vi "Re-Start Measurement.vi"(8 "error in (no error)":errorcluster, 11 "Spectrum Recorder too in":refnum<class "Spectrum Recorder too.lvclass">) -> (0 "error out":errorcluster, 3 "Spectrum Recorder too out":refnum<class "Spectrum Recorder too.lvclass">)   [LabVIEW 2018, in "Spectrum Recorder too.lvclass"]
uses:
  Spectrum Recorder too.lvclass
  C:/github/2018/LabActor/Instrument Actor/Instrument Actor.lvclass
  Spectrum Recorder too.lvclass/Spectrum Recorder too.ctl
  Instrument Actor/Instrument Actor.lvclass/Instrument Actor.ctl
  Instrument Actor/Read Instrument driver.vi
  Instrument Actor/Write Instrument driver.vi
  NHMFL_Core/Libraries/Instruments/Instrument Driver/Instrument Driver.lvclass
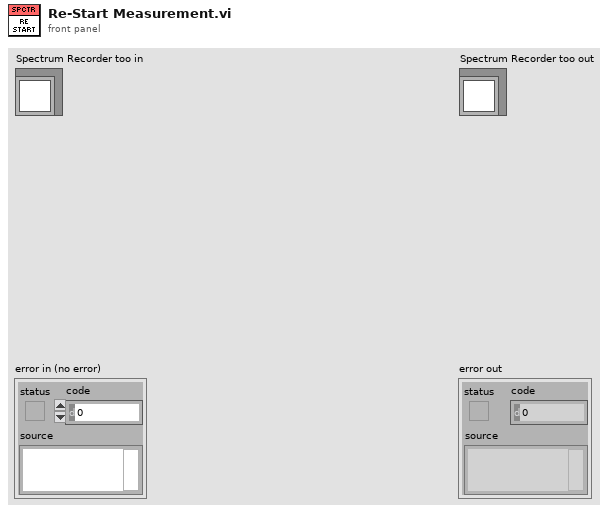
[diagram p1: front panel]
types:
  T1 = enum16{"open", "replace", "create", "open or create", "replace or create", "replace or create with confirmation"}
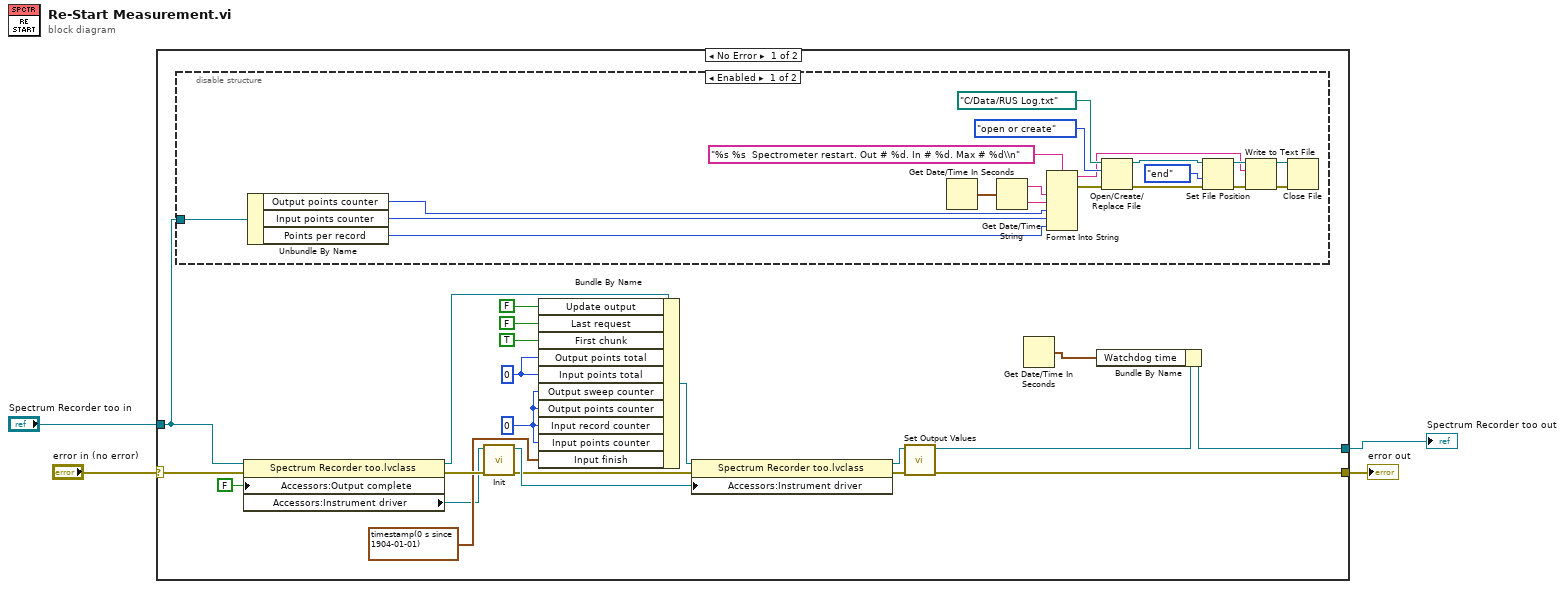
[diagram p0: block diagram]
diagram:
  n1 = case shown="No Error" "error in (no error)" {
    selector: "error in (no error)" -> [w15 w46]
    tunnel: [w10 w46] -> w3
    tunnel: [w6 w45] -> w1
    tunnel: "Spectrum Recorder too in" -> [w7 w45]
    frame No Error {
      w20 = i64 0 ("Output points total")
      w18 = 0 ("Output sweep counter")
      n2 = disable-structure shown="Enabled" {
        disable-tunnel: w7 -> [w29 _]
        frame Enabled {
          n3 = Unbundle By Name(w29) -> ("Output points counter"=w28:i32, "Input points counter"=w27:i32, "Points per record"=w26:i32)
          n4 = Get Date/Time In Seconds() -> (seconds since 1Jan1904=w34:timestamp)
          n5 = Get Date/Time String(seconds (now)=w34) -> (date string=w33:string, time string=w32:string)  [unwired: 2 in]
          n6 = Format Into String(format string="%s %s  Spectrometer restart. Out # %d. In # %d. Max # %d\\n", w33, w32, w28, w27, w26) -> (resulting string=w31:string, error out=w30:errorcluster)  [unwired: 2 in]
          n7 = Open/Create/Replace File(file path (use dialog)=path "C:/Data/RUS Log.txt" ("file (use dialog)"), error in=w30, operation (0:open)=T1."open or create") -> (refnum out=w42:refnum<file>, error out=w39:errorcluster)  [unwired: 3 in, 1 out]
          n8 = Set File Position(refnum=w42, from (0:start)=enum16{"start", "end", "current"}."end", error in=w39) -> (refnum out=w41:refnum<file>, error out=w38:errorcluster)  [unwired: 1 in]
          n9 = Write to Text File(file (use dialog)=w41, text=w31, error in=w38) -> (refnum out=w36:refnum<file>, error out=w37:errorcluster)  [unwired: 1 in, 1 out]
          n10 = Close File(refnum=w36, error in=w37) -> ()  [unwired: 2 out]
        }
        frame Disabled {
        }
      }
      n11 = property class="Spectrum Recorder too.lvclass"(reference=w7, error in=w15, "Accessors:Output complete"=FALSE ("Output complete")) -> (reference out=w8:refnum<class "Spectrum Recorder too.lvclass">, error out=w24:errorcluster, "Accessors:Instrument driver"=w17:refnum<class "Instrument Driver.lvclass">)
      n12 = call-dynamic "Init.vi"("error in (no error)"=w24, "Instrument Driver in"=w17) -> ("error out"=w12:errorcluster, "Instrument Driver out"=w16:refnum<class "Instrument Driver.lvclass">)  [unwired: 7 in, 1 out]
      n13 = Bundle By Name(cluster=w8, "Update output"=FALSE, "Last request"=FALSE, "First chunk"=TRUE, "Output points total"=w20, "Input points total"=w20, "Output sweep counter"=w18, "Output points counter"=w18, "Input record counter"=w18, "Input points counter"=w18, "Input finish"=timestamp(0 s since 1904-01-01)) -> (w14:refnum<class "Spectrum Recorder too.lvclass">)
      n14 = property class="Spectrum Recorder too.lvclass"(reference=w14, error in=w12, "Accessors:Instrument driver"=w16) -> (reference out=w13:refnum<class "Spectrum Recorder too.lvclass">, error out=w11:errorcluster)
      n15 = call-dynamic "Set Output Values.vi"("error in (no error)"=w11, "Spectrum Recorder in"=w13) -> ("error out"=w10:errorcluster, "Spectrum Recorder out"=w9:refnum<class "Spectrum Recorder too.lvclass">)  [unwired: 8 in]
      n16 = Get Date/Time In Seconds() -> (seconds since 1Jan1904=w5:timestamp)
      n17 = Bundle By Name(cluster=w9, "Watchdog time"=w5) -> (w6:refnum<class "Spectrum Recorder too.lvclass">)
    }
    frame Error {
    }
  }
  "error out" <- w3
  "Spectrum Recorder too out" <- w1
